vi "CPP_Aeroprobe.vi"() -> (5 "Plug in titles":string[](array[string]), 7 "Plug in values":string[](array[string]))   [LabVIEW 2012]
uses:
  Globals/Meas_global.vi
  Globals/Trav_pos_global.vi
panel:
  in  "Mode":enum32{"Measure", "Take Zeroes"}(radio)=enum."Take Zeroes"
  in  "RunManually?":bool
  in  "Old5HoleProbe?":bool
  out "return type":i32
  out "p-p0":dbl[](array[numeric]) format="%#.5f"
  out "Temperature/C":dbl format="%#.1f"
  out "Pressure/mBar":dbl
  out "timeOfzero":timestamp
  out "zeroShift/mmH2O":dbl[](array[numeric]) format="%#.6f"
  out "Velocity":dbl
  out "W":dbl
  out "V":dbl
  out "U":dbl caption="u  m/s"
  # "!! 5-hole 1-5 must be connected to Channels 1-5 !!"
  # "Zero Info"
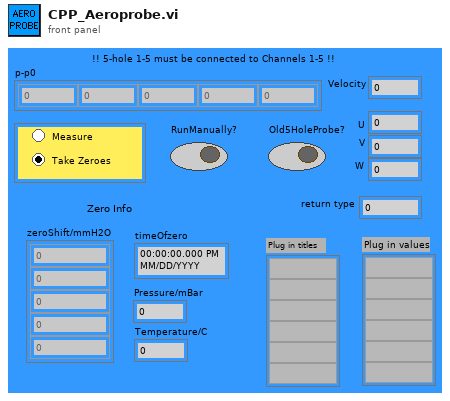
[diagram p1: front panel]
types:
  T1 = typedef "Post_Process.ctl" = enum16{"Take New Data", "Post Process Raw Data File"}
  T2 = typedef "Traverse_cluster.ctl" = cluster{"Start X":dbl, "Start Y":dbl, "Start Z":dbl, "End X":dbl, "End Y":dbl, "End Z":dbl, "No. of pts.":i32, "Spacing":T3, "Filename":path, "Tunnel Speed":dbl, "Averaging time (min)":dbl, "Extra Commands":string, "Specific Arguments":string, "Emission Rate (l/min)":dbl, "Trace Gas Concentration (%)":dbl, "Density Ratio":string, "Comments":string, "Row No":i32, "Row Type Selector":T4, "Completion time":string, "Row Duration (mins)":dbl, "No. of Valid pts.":i32, "Meas Setup File":string}
  T3 = typedef "Spacing.ctl" = enum16{"Linear", "Log", "Gauss", "Specified", "N/A"}
  T4 = typedef "Multi_run_mode.ctl" = enum16{"Move Traverse Only", "Set Tunnel Speed Only", "Set Source Only", "Set Measurement Conditions", "Single Measurement", "Vertical Profile", "Lateral Profile", "Longitudinal Profile", "Explore Volume", "Multi-Axis Profile", "Auto Calibrate", "Meas Fast FID Bkgnd", "Check Beam Power", "Scanning Valve Measurement", "Run VI Named:", "Set ADAM Ch", "Wait (minutes)", "Send Message", "Synchronize With:", "Fall Back to this Row", "Turn Off Row Repeating", "Blank Row", "Traverse 3D Volume"}
  T5 = typedef "Analysis_info_cluster.ctl" = cluster{"Colour":u32, "Inst type":T6, "Inst name":string, "Symbol":string, "Code name":string, "Extra Info":string, "Inst Array":T7, "Extra Titles":string[], "Extra Values":string[], "U":dbl, "u^2":dbl, "u^3":dbl, "u^4":dbl, "Skew_u":dbl, "Kurt_u":dbl, "Sd Error in Mean":dbl, "% u'/U":dbl, "X":dbl, "Y":dbl, "Z":dbl, "Timescale integral to 25%":dbl, "Sd Error in Variance":dbl, "Calib File":path, "Calib Constants":dbl[], "Output Position":bool, "Full Stats":bool, "Av Sampling Rate":dbl, "Av No of Samples":dbl, "Total Meas Time (s)":dbl, "ADAM Ch Name":string}
  T6 = typedef "Inst_type.ctl" = enum16{"Propeller anemometer", "Raw voltage", "Pressure Transducer", "Pitot-static tube", "Preston tube", "Hot wire", "Cross wire 1", "Cross wire 2", "Generic Linear", "Generic Polynomial", "Generic BackPoly", "Fast FID", "Thermocouple", "Cold wire", "Pulsed Wire", "LDA Vel", "LDA Tran time", "LDA Arr time"}
  T7 = typedef "Instrument_Array.ctl" = enum16{"PWA", "LDA", "Analogue"}
  T8 = cluster{"Analysis Info cluster[0]":T5, "Analysis Info cluster[1]":T5, "Analysis Info cluster[2]":T5, "Analysis Info cluster[3]":T5, "Analysis Info cluster[4]":T5, "Analysis Info cluster[5]":T5, "Analysis Info cluster[6]":T5}
  T9 = cluster{"Analysis Info cluster[0]":T5, "Analysis Info cluster[1]":T5, "Analysis Info cluster[2]":T5, "Analysis Info cluster[3]":T5, "Analysis Info cluster[4]":T5, "Analysis Info cluster[5]":T5, "Analysis Info cluster[6]":T5, "Analysis Info cluster[7]":T5, "Analysis Info cluster[8]":T5, "Analysis Info cluster[9]":T5, "Analysis Info cluster[10]":T5, "Analysis Info cluster[11]":T5, "Analysis Info cluster[12]":T5, "Analysis Info cluster[13]":T5}
  T10 = cluster{"[0]":dbl, "[1]":dbl, "[2]":dbl, "[3]":dbl, "[4]":dbl}
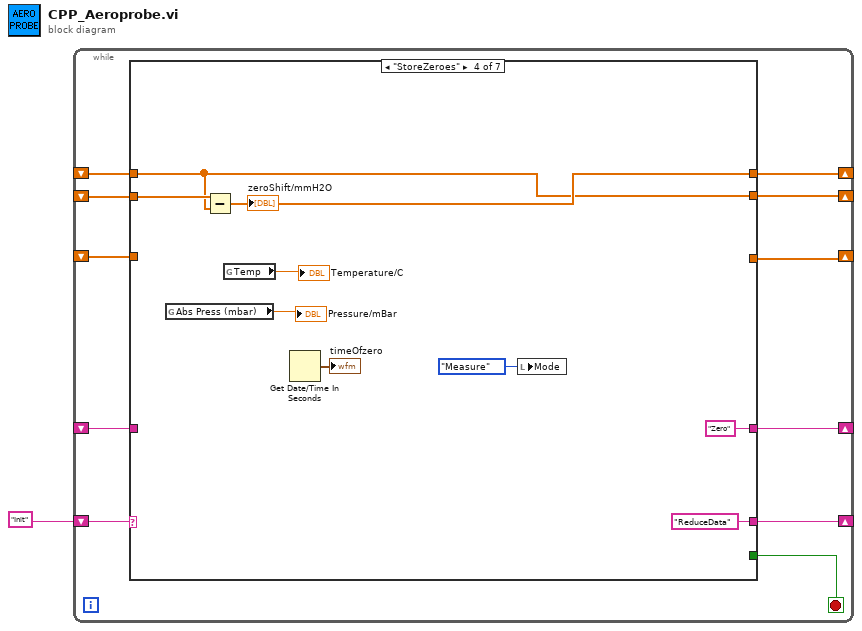
[diagram p0: block diagram]
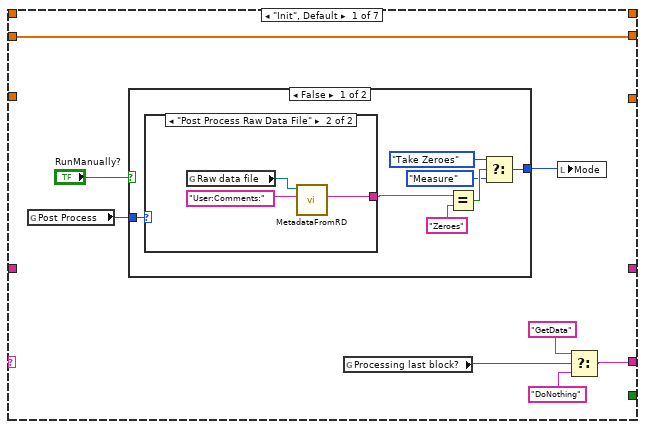
[diagram p2: hidden frame]
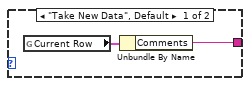
[diagram p3: hidden frame]
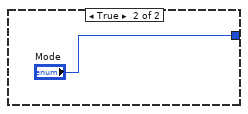
[diagram p4: hidden frame]
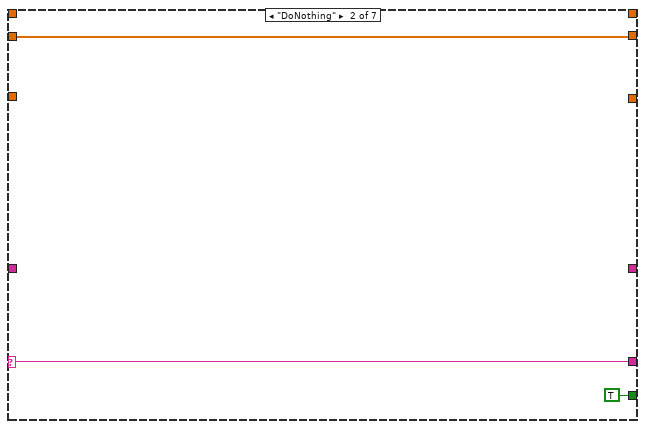
[diagram p5: hidden frame]
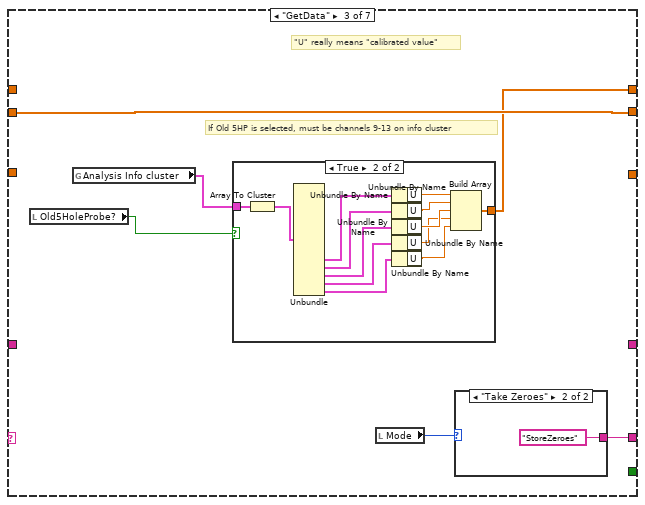
[diagram p6: hidden frame]
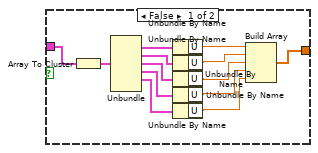
[diagram p7: hidden frame]
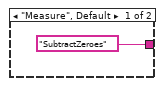
[diagram p8: hidden frame]
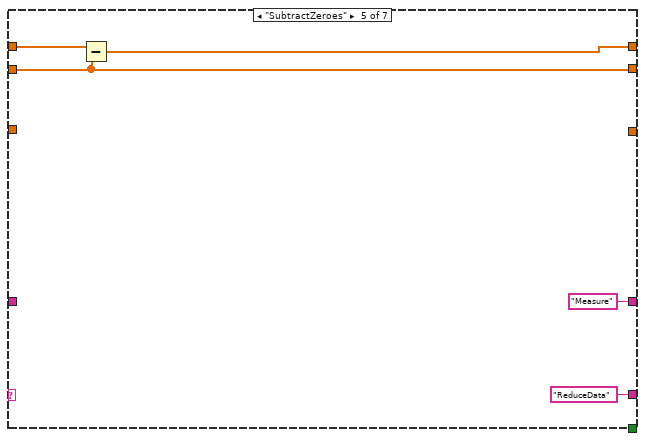
[diagram p9: hidden frame]
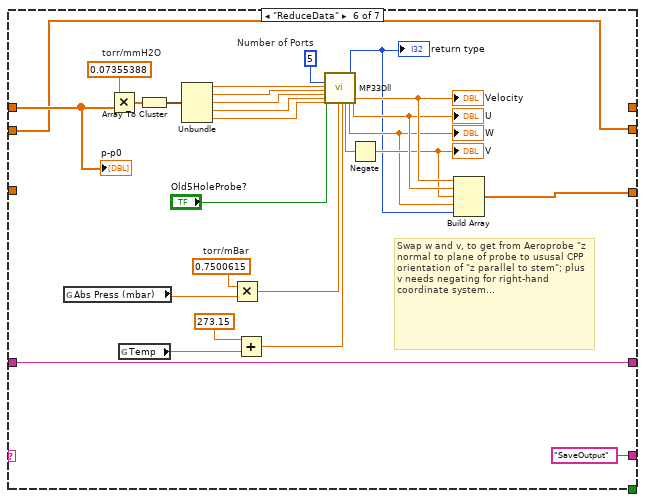
[diagram p10: hidden frame]
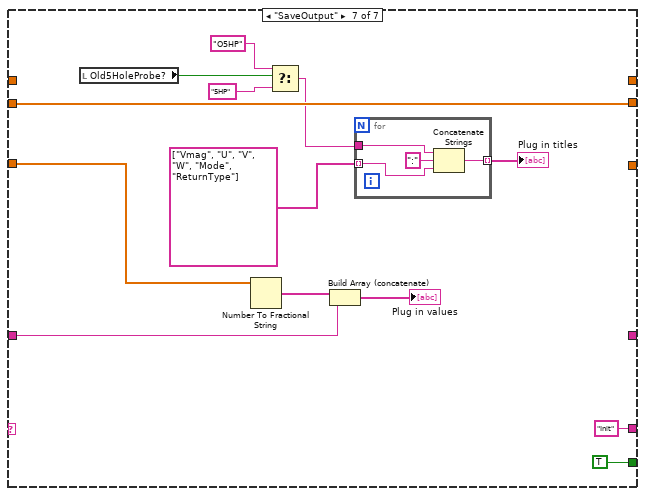
[diagram p11: hidden frame]
diagram:
  n1 = while {
    shift-right: [w11] -> _
    shift-left: "Init" -> [w12]
    shift-right: [w10] -> _
    shift-left: _ -> [w8]
    shift-right: [w9] -> _
    shift-left: _ -> [w7]
    shift-right: [w6] -> _
    shift-left: _ -> [w5]
    shift-right: [w3] -> _
    shift-left: _ -> [w2]
    stop <- w4 stop-if-true
    n2 = case shown="\"StoreZeroes\"" w12 {
      selector: w12 -> [_ w36 _ _ _ _ _]
      tunnel: [w20 w36 w42 "ReduceData" "ReduceData" "SaveOutput" "Init"] -> w11
      tunnel: [_ _ w38 w77 w83 _ _] -> w10
      tunnel: [w16 w34 w41 w71 w82 w96 w124] -> w9
      tunnel: w8 -> [_ _ _ w71 w84 w105 _]
      tunnel: w7 -> [w16 w34 w41 w79 w82 w96 w124]
      tunnel: [_ _ _ _ _ w92 _] -> w6
      tunnel: w5 -> [_ _ _ _ _ _ w123]
      tunnel: [_ TRUE _ _ _ _ TRUE] -> w4
      tunnel: [_ _ _ "Zero" "Measure" w91 _] -> w3
      tunnel: w2 -> [_ _ _ _ _ w91 w118]
      frame "Init", Default {
        n3 = global read "Meas_global.vi" "Post Process"() -> (w13:T1)
        n4 = case shown="False" "RunManually?" {
          tunnel: [w27 "Mode"] -> w14
          tunnel: w13 -> [w21 _]
          frame False {
            n5 = case shown="\"Post Process Raw Data File\"" w21 {
              tunnel: [w28 w30] -> w26
              frame "Take New Data", Default {
                n6 = global read "Trav_pos_global.vi" "Current Row"() -> (w29:T2)
                n7 = Unbundle By Name(w29) -> ("Comments"=w28:string)
              }
              frame "Post Process Raw Data File" {
                n8 = global read "Meas_global.vi" "Raw data file"() -> (w32:path)
                n9 = call "MetadataFromRD.vi"("ChannelName"="User:Comments:", "Raw data file"=w32) -> ("ValueString"=w30:string)  [unwired: 8 in, 1 out]
              }
            }
            n10 = Equal?(x=w26, y="Zeroes") -> (x = y?=w24:bool)
            n11 = Select(t=enum32{"Measure", "Take Zeroes"}."Take Zeroes" ("Mode"), s=w24, f=enum32{"Measure", "Take Zeroes"}."Measure" ("Mode")) -> (s? t:f=w27:enum32{"Measure", "Take Zeroes"})
          }
          frame True {
          }
        }
        n12 = global read "Meas_global.vi" "Processing last block?"() -> (w19:bool)
        n13 = local write "Mode"(w14) -> ()
        n14 = Select(t="GetData", s=w19, f="DoNothing") -> (s? t:f=w20:string)
      }
      frame "DoNothing" {
      }
      frame "GetData" {
        # "If Old 5HP is selected, must be channels 9-13 on info cluster"
        # "\"U\" really means \"calibrated value\""
        n15 = local read "Old5HoleProbe?"() -> (w40:bool)
        n16 = global read "Meas_global.vi" "Analysis Info cluster"() -> (w39:T5[])
        n17 = case shown="True" w40 {
          tunnel: w39 -> [w44 w64]
          tunnel: [w43 w58] -> w38
          frame False {
            n18 = Array To Cluster(array=w44) -> (cluster=w50:T8)
            n19 = Unbundle(w50) -> ("Analysis Info cluster[1]"=w49:T5, "Analysis Info cluster[2]"=w48:T5, "Analysis Info cluster[3]"=w47:T5, "Analysis Info cluster[4]"=w46:T5, "Analysis Info cluster[5]"=w45:T5)  [unwired: 2 out]
            n20 = Unbundle By Name(w49) -> ("U"=w51:dbl)
            n21 = Unbundle By Name(w48) -> ("U"=w52:dbl)
            n22 = Unbundle By Name(w47) -> ("U"=w53:dbl)
            n23 = Unbundle By Name(w46) -> ("U"=w54:dbl)
            n24 = Unbundle By Name(w45) -> ("U"=w55:dbl)
            n25 = Build Array(w51, w52, w53, w54, w55) -> (w43:dbl[])
          }
          frame True {
            n26 = Array To Cluster(array=w64) -> (cluster=w65:T9)
            n27 = Unbundle(w65) -> ("Analysis Info cluster[9]"=w63:T5, "Analysis Info cluster[10]"=w62:T5, "Analysis Info cluster[11]"=w61:T5, "Analysis Info cluster[12]"=w60:T5, "Analysis Info cluster[13]"=w59:T5)  [unwired: 9 out]
            n28 = Unbundle By Name(w63) -> ("U"=w66:dbl)
            n29 = Unbundle By Name(w62) -> ("U"=w67:dbl)
            n30 = Unbundle By Name(w61) -> ("U"=w57:dbl)
            n31 = Unbundle By Name(w60) -> ("U"=w56:dbl)
            n32 = Unbundle By Name(w59) -> ("U"=w68:dbl)
            n33 = Build Array(w66, w67, w57, w56, w68) -> (w58:dbl[])
          }
        }
        n34 = local read "Mode"() -> (w37:enum32{"Measure", "Take Zeroes"})
        n35 = case shown="\"Take Zeroes\"" w37 {
          tunnel: ["SubtractZeroes" "StoreZeroes"] -> w42
          frame "Measure", Default {
          }
          frame "Take Zeroes" {
          }
        }
      }
      frame "StoreZeroes" {
        n36 = global read "Meas_global.vi" "Abs Press (mbar)"() -> (→"Pressure/mBar":dbl)
        n37 = Subtract(x=w79, y=w71) -> (x-y=w77:dbl[])
        "zeroShift/mmH2O" <- w77
        n38 = global read "Meas_global.vi" "Temp"() -> (→"Temperature/C":dbl)
        n39 = Get Date/Time In Seconds() -> (seconds since 1Jan1904=→"timeOfzero":timestamp)
        n40 = local write "Mode"(enum32{"Measure", "Take Zeroes"}."Measure" ("Mode")) -> ()
      }
      frame "SubtractZeroes" {
        n41 = Subtract(x=w84, y=w82) -> (x-y=w83:dbl[])
      }
      frame "ReduceData" {
        w106 = 0.07355388  # torr/mmH2O
        w110 = 0.7500615  # torr/mBar
        w107 = 5  # Number of Ports
        # "Swap w and v, to get from Aeroprobe \"z normal to plane of probe to ususal CPP orientation of \"z parallel to stem\"; plus v needs negating for right-hand coordinate system..."
        n42 = global read "Meas_global.vi" "Abs Press (mbar)"() -> (w87:dbl)
        n43 = Multiply(x=w106, y=w105) -> (x*y=w104:dbl[])
        n44 = global read "Meas_global.vi" "Temp"() -> (w88:dbl)
        n45 = Array To Cluster(array=w104) -> (cluster=w103:T10)
        n46 = Unbundle(w103) -> ("[0]"=w102:dbl, "[1]"=w101:dbl, "[2]"=w100:dbl, "[3]"=w99:dbl, "[4]"=w98:dbl)
        n47 = Multiply(x=w110, y=w87) -> (x*y=w109:dbl)
        n48 = Add(x=273.15, y=w88) -> (x+y=w111:dbl)
        n49 = call "MP33Dll.vi"("Old5HoleProbe?"="Old5HoleProbe?", "Number of Ports"=w107, "P1 Torr"=w102, "P2 Torr"=w101, "P3 Torr"=w100, "P4 Torr"=w99, "P5 Torr"=w98, "Pref Torr"=w109, "TTot Kelvin"=w111) -> ("w m/s"=w93:dbl, "return type"=w86:i32, "v m/s"=w89:dbl, "VMagn m/s"=w95:dbl, "u  m/s"=w94:dbl)  [unwired: 8 in, 6 out]
        "U" <- w94
        "W" <- w89
        "Velocity" <- w95
        "return type" <- w86
        n50 = Negate(x=w93) -> (-x=w90:dbl)
        "V" <- w90
        n51 = Build Array(w95, w94, w90, w89, w86) -> (w92:dbl[])
        "p-p0" <- w105
      }
      frame "SaveOutput" {
        n52 = local read "Old5HoleProbe?"() -> (w116:bool)
        n53 = Number To Fractional String(number=w123) -> (F-format string=w122:string[])  [unwired: 3 in]
        n54 = Select(t="O5HP", s=w116, f="5HP") -> (s? t:f=w113:string)
        n55 = Build Array (concatenate)(w122, w118) -> (→"Plug in values":string[])
        n56 = for {
          tunnel: string[] ["Vmag", "U", "V", "W", "Mode", "ReturnType"] ("Plug in titles") -> [w126] mode=indexing
          tunnel: w113 -> [w128]
          tunnel: [w125] -> w112 mode=indexing
          n57 = Concatenate Strings(w128, ":" ("string"), w126) -> (w125:string)
        }
        "Plug in titles" <- w112
      }
    }
  }
